vi "Listen for Interrupt.vi"(8 "error in (no error)":errorcluster, 10 "Response Msg in":refnum<class "Response Msg.lvclass">, 11 "Response Core in":refnum<class "Response Core.lvclass">) -> (0 "error out":errorcluster, 2 "Response Msg out":refnum<class "Response Msg.lvclass">, 3 "Response Core out":refnum<class "Response Core.lvclass">)   [LabVIEW 2020, in "Publisher.lvlib" / "Response Core.lvclass"]
doc: "Await interrupt in parallel with recieve to enable termination of Recieve.\n\nThe default implementation does nothing."
uses:
  Response Core.lvclass
  Response Msg.lvclass
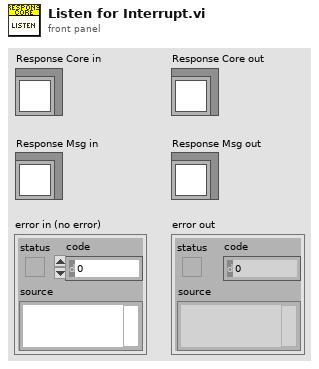
[diagram p1: front panel]
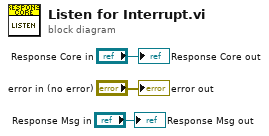
[diagram p0: block diagram]
diagram:
  "error out" <- "error in (no error)"
  "Response Core out" <- "Response Core in"
  "Response Msg out" <- "Response Msg in"
